vi "Evaluate Part 1.vi"() -> ()   [LabVIEW 2021]
uses:
  Proto/Rule.lvclass
panel:
  out "sum":i32
  in  "Input":string="px{a<2006:qkq,m>2090:A,rfg}\npv{a>1716:R,A}\nlnx{m>1548:A,A}\nrfg{s<537:gd,x>2440:R,A}\nqs{s>3448:A,lnx}\nqkq{x<1416:A,crn}\ncrn{x>2662:A,R}\nin{s<1351:px,qqz}\nqqz{s>2770:qs,m<1801:hdj,R}\ngd{a>3333:R,R}\nhdj{m>838:A,pv}\n\n{x=787,m=2655,a=1222,s=2876}\n{x=1679,m=44,a=2067,s=496}\n{x=2036,m=264,a=79,s=2244}\n{x=2461,m=1339,a=466,s=291}\n{x=2127,m=1623,a=2188,s=1013}"
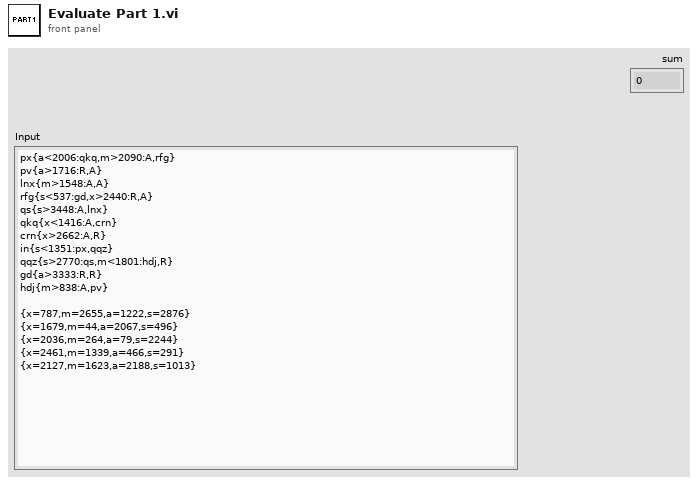
[diagram p1: front panel]
types:
  T1 = cluster{"[0]":i32, "[1]":i32, "[2]":i32, "[3]":i32}[]
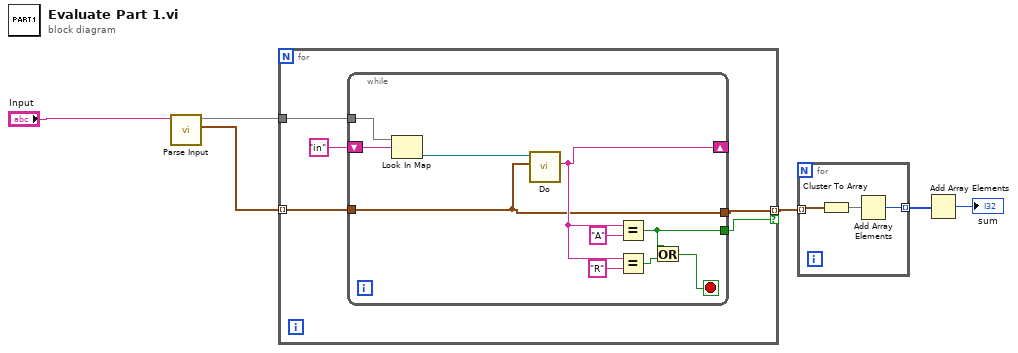
[diagram p0: block diagram]
diagram:
  n1 = call "Parse Input.vi"("Input"="Input") -> ("Array"=w4:T1, "map"=w5:map{string, refnum<class "Rule.lvclass">})  [unwired: 9 in]
  n2 = for {
    tunnel: w5 -> [w9]
    tunnel: w4 -> [w10] mode=indexing
    tunnel: [w8] -> w3 mode=indexing if=w7
    n3 = while {
      shift-right: [w17] -> _
      shift-left: "in" ("key") -> [w21]
      tunnel: w10 -> [w13]
      tunnel: w9 -> [w20]
      tunnel: [w13] -> w8
      tunnel: [w12] -> w7
      stop <- w14 stop-if-true
      n4 = Look In Map(map=w20, key=w21) -> (value=w19:refnum<class "Rule.lvclass">)  [unwired: 1 in, 1 out]
      n5 = call "Do.vi"("Cluster"=w13, "Proto in"=w19) -> ("Label"=w17:string)  [unwired: 7 in, 2 out]
      n6 = Equal?(x=w17, y="A") -> (x = y?=w12:bool)
      n7 = Equal?(x=w17, y="R") -> (x = y?=w15:bool)
      n8 = Or(x=w12, y=w15) -> (x .or. y?=w14:bool)
    }
  }
  n9 = for {
    tunnel: w3 -> [w24] mode=indexing
    tunnel: [w22] -> w2 mode=indexing
    n10 = Cluster To Array(cluster=w24) -> (array=w23:i32[])
    n11 = Add Array Elements(numeric array=w23) -> (sum=w22:i32)
  }
  n12 = Add Array Elements(numeric array=w2) -> (sum=→"sum":i32)
